vi "pic_step1.vi"() -> ()   [LabVIEW 2018]
uses:
  Device VIs/Verbal.vi
  <vilib>/Instr/_visa.llb/VISA Configure Serial Port (Instr).vi
panel:
  in  "结束":bool
  out "P3右":bool
  out "P2 右":bool
  out "P1 右":bool
  out "pic3Left":bool caption="0位"
  out "pic3Right":bool caption="限位"
  out "pic2Left":bool caption="0位"
  out "pic2Right":bool caption="限位"
  out "pic1Left":bool caption="0位"
  out "pic1Right":bool caption="限位"
  out "CH3 当前位置":i32
  in  "P3jog":bool caption="X jog"
  out "P3设定位置":i32
  in  "pic3位置":u16(ring) caption="位置" items=["位置0", "位置1", "位置2", "位置3"]
  in  "P3归0":bool
  in  "CH3启动":bool
  in  "CH3 运动步数":i32 caption="P3 步进"
  in  "Y 连续正转":bool
  in  "X连续反转":bool
  out "Yflag":bool
  out "0位":u8
  in  "P2 jog":bool caption="X jog"
  in  "P1jog":bool caption="X jog"
  in  "Zjog":bool caption="X jog"
  in  "Yjog":bool caption="X jog"
  in  "X jog":bool
  out "P2设定位置":i32
  out "P1设定位置":i32
  out "Z设定位置":i32
  out "Y设定位置":i32
  out "X设定位置":i32
  in  "pic2位置":u16(ring) caption="位置" items=["位置0", "位置1", "位置2", "位置3"]
  in  "pic1位置":u16(ring) caption="位置" items=["位置0", "位置1", "位置2", "位置3"]
  in  "Z轴位置":u16(ring) caption="位置" items=["位置0", "位置1", "位置2", "位置3"]
  in  "Y轴位置":u16(ring) caption="位置" items=["位置0", "位置1", "位置2", "位置3"]
  in  "X轴位置":u16(ring) caption="位置" items=["位置0", "位置1", "位置2", "位置3"]
  out "执行":bool
  in  "Z 归0":bool
  in  "Y 归0":bool
  in  "X 归0":bool
  out "当前位置":string[](array[string])
  in  "Z 连续反转":bool
  in  "Z 连续正转":bool
  in  "Y 连续反转":bool
  in  "X 连续正转":bool
  out "Z Left":bool caption="0位"
  out "Z Right":bool caption="限位"
  out "Y Left":bool caption="0位"
  out "Y Right":bool caption="限位"
  out "X Lift":bool caption="0位"
  out "X Right":bool caption="限位"
  in  "Z 启动":bool
  in  "Y 启动":bool
  in  "X 启动":bool
  in  "Step Z":i32 caption="Z 步进" min=-8388607 max=8388607
  in  "Step Y":i32 caption="Y 步进" min=-8388607 max=8388607
  in  "Step X":i32 caption="X 步进" min=-8388607 max=8388607
  in  "P2归0":bool
  in  "P1 归0":bool
  out "OK":bool
  in  "制动":bool
  in  "CH2启动":bool
  in  "CH1启动":bool
  in  "CH2 运动步数":i32 caption="P2 步进"
  in  "CH1 运动步数":i32 caption="P1 步进"
  out "CH2 当前位置":i32
  out "CH1 当前位置":i32
  out "状态":string
  out "error out":errorcluster
  # "X"
  # "Y"
  # "Z"
  # "P1"
  # "P2"
  # "P3"
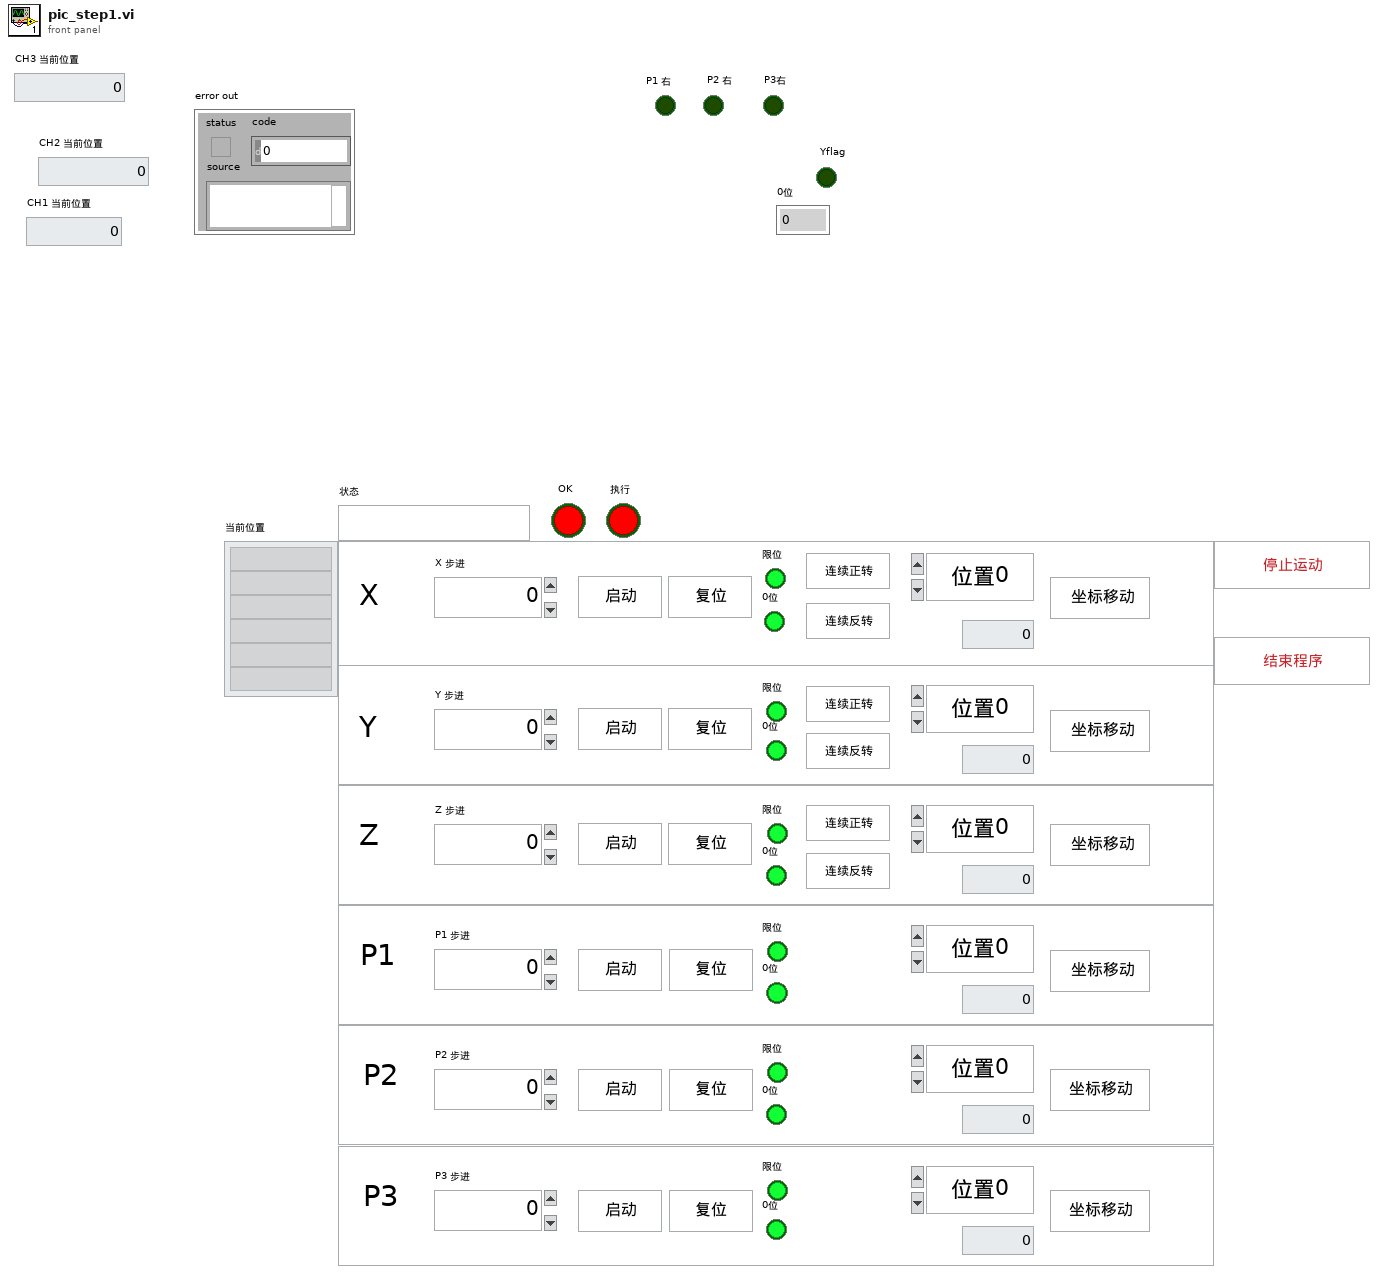
[diagram p1: front panel]
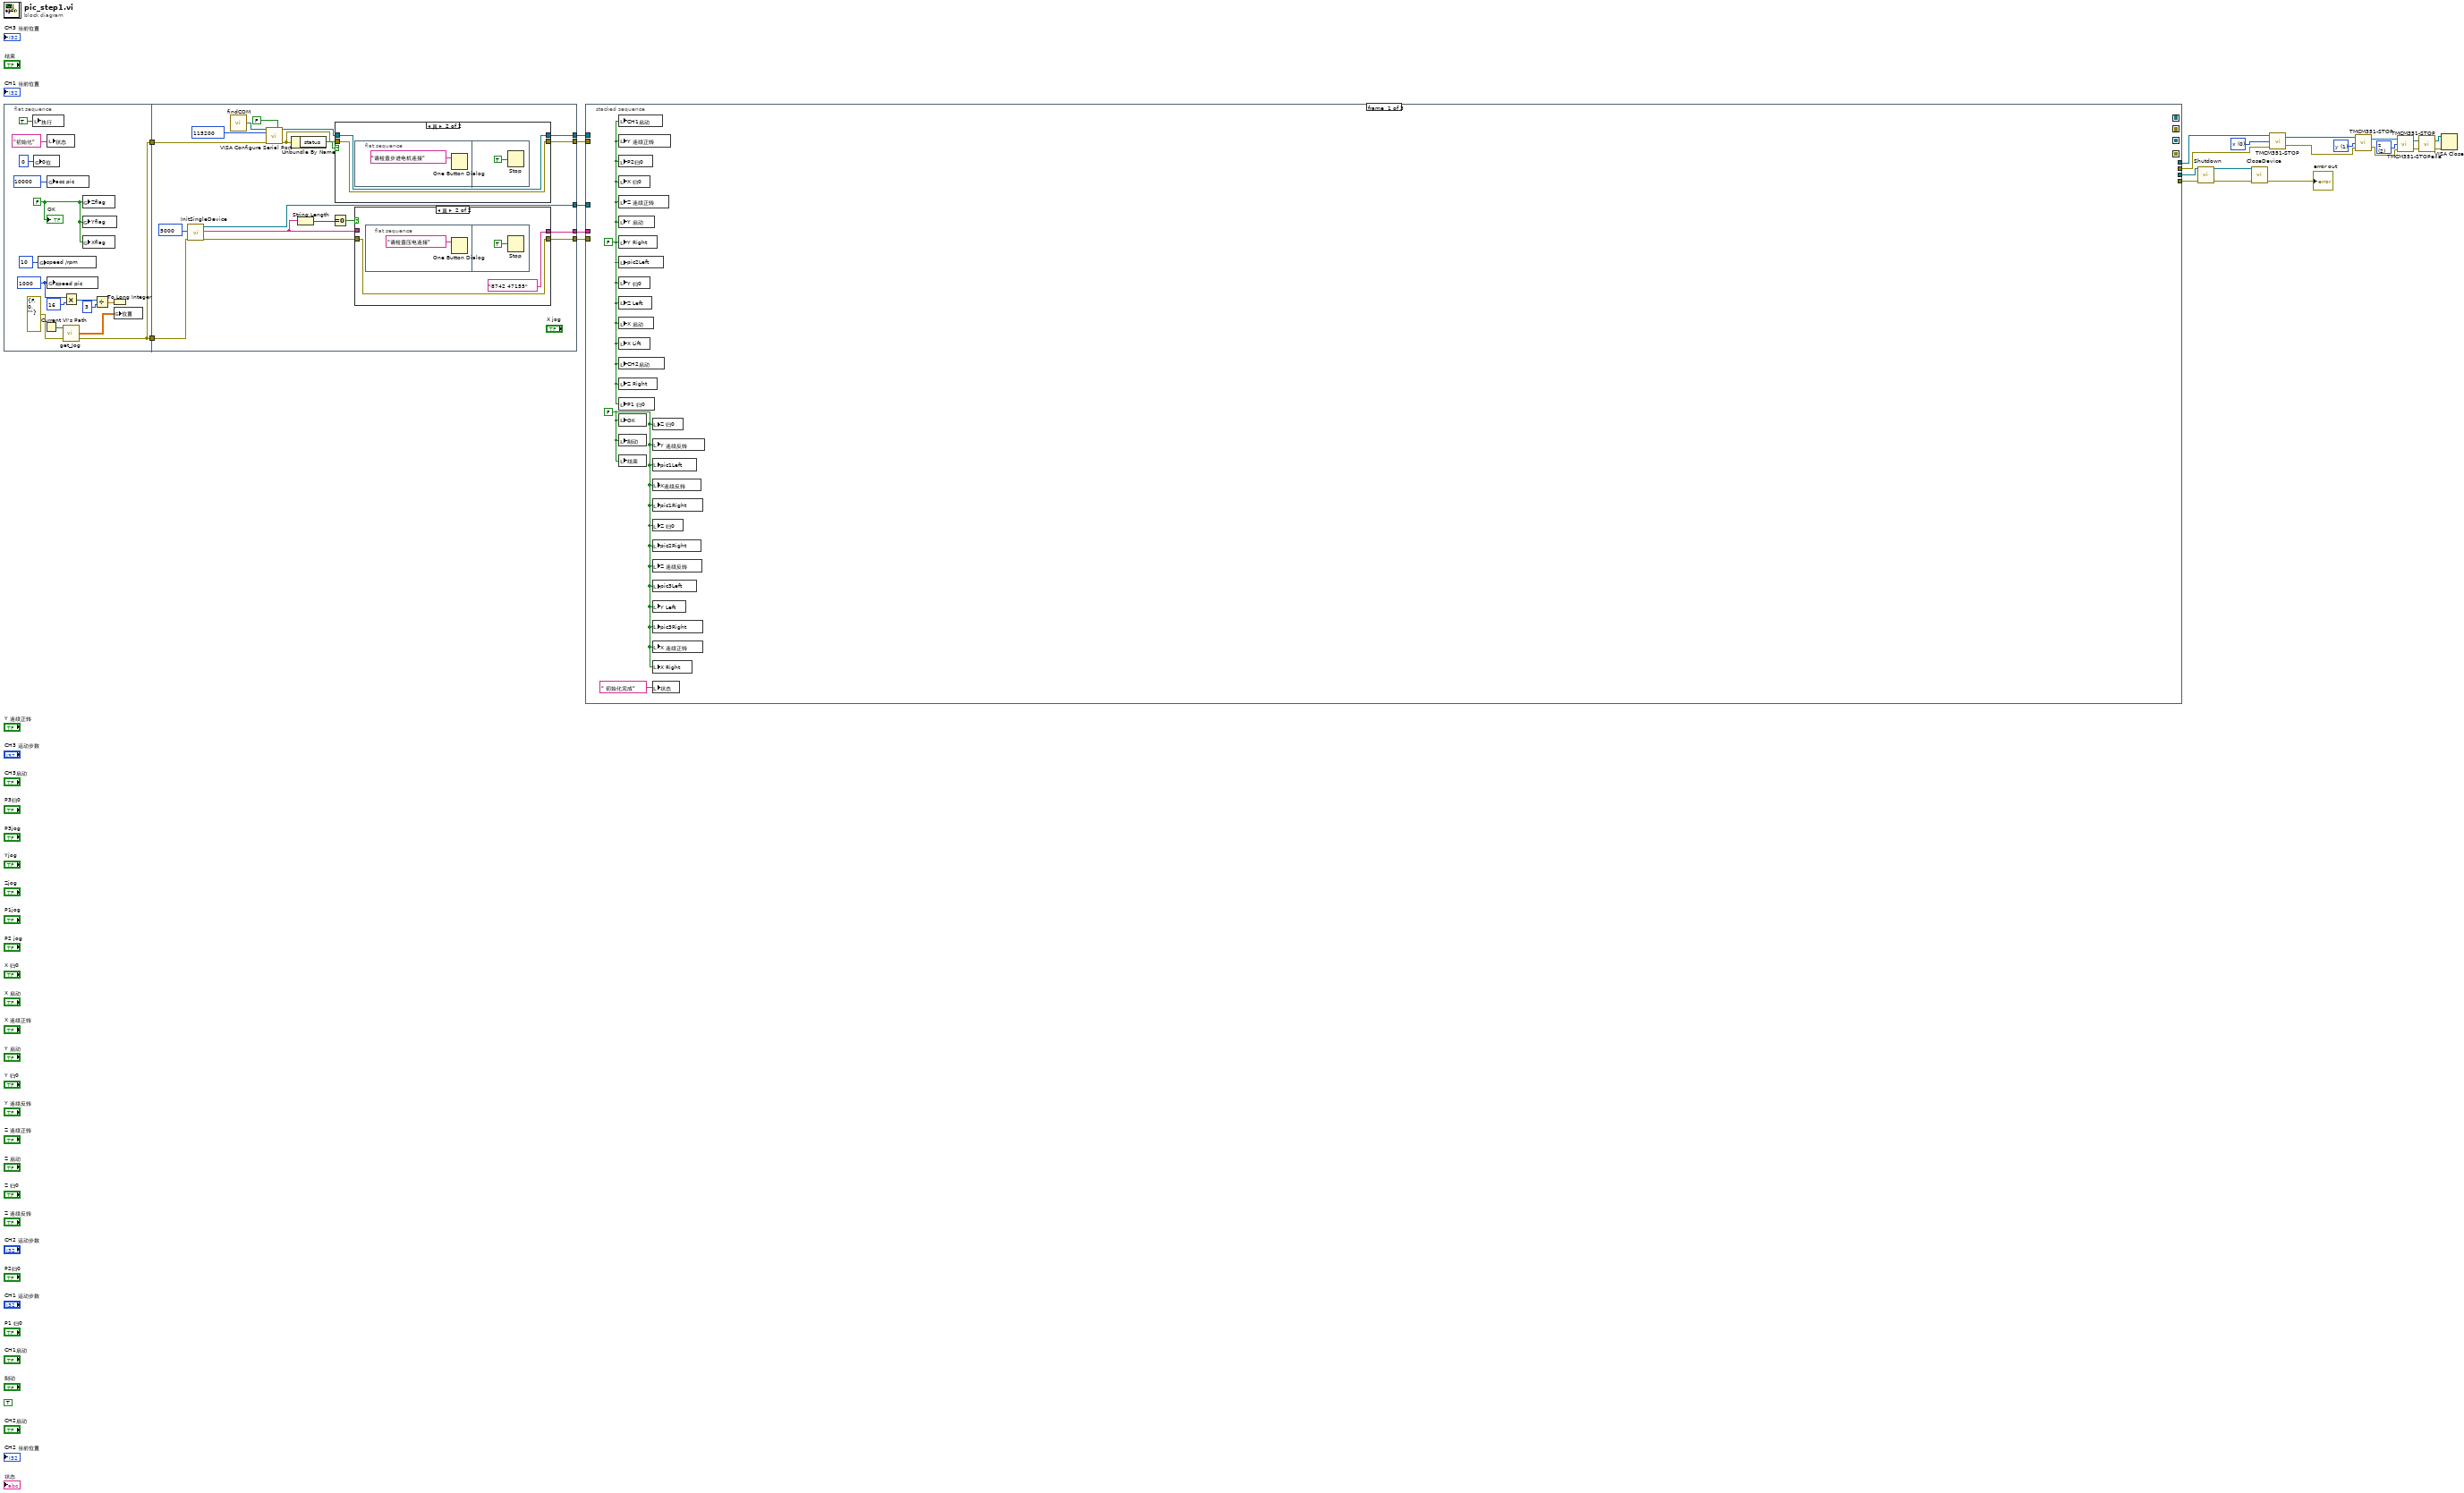
[diagram p0: block diagram]
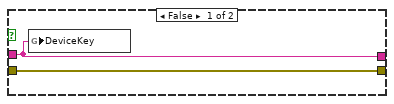
[diagram p2: hidden frame]
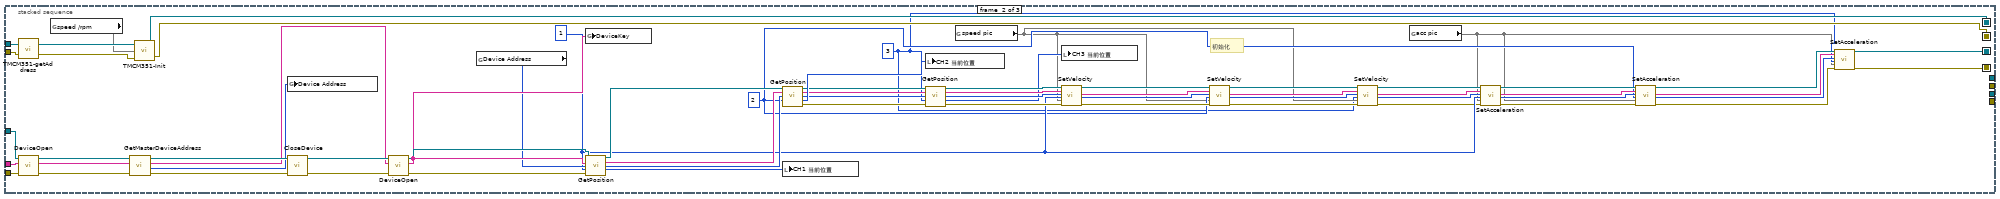
[diagram p4: hidden frame]
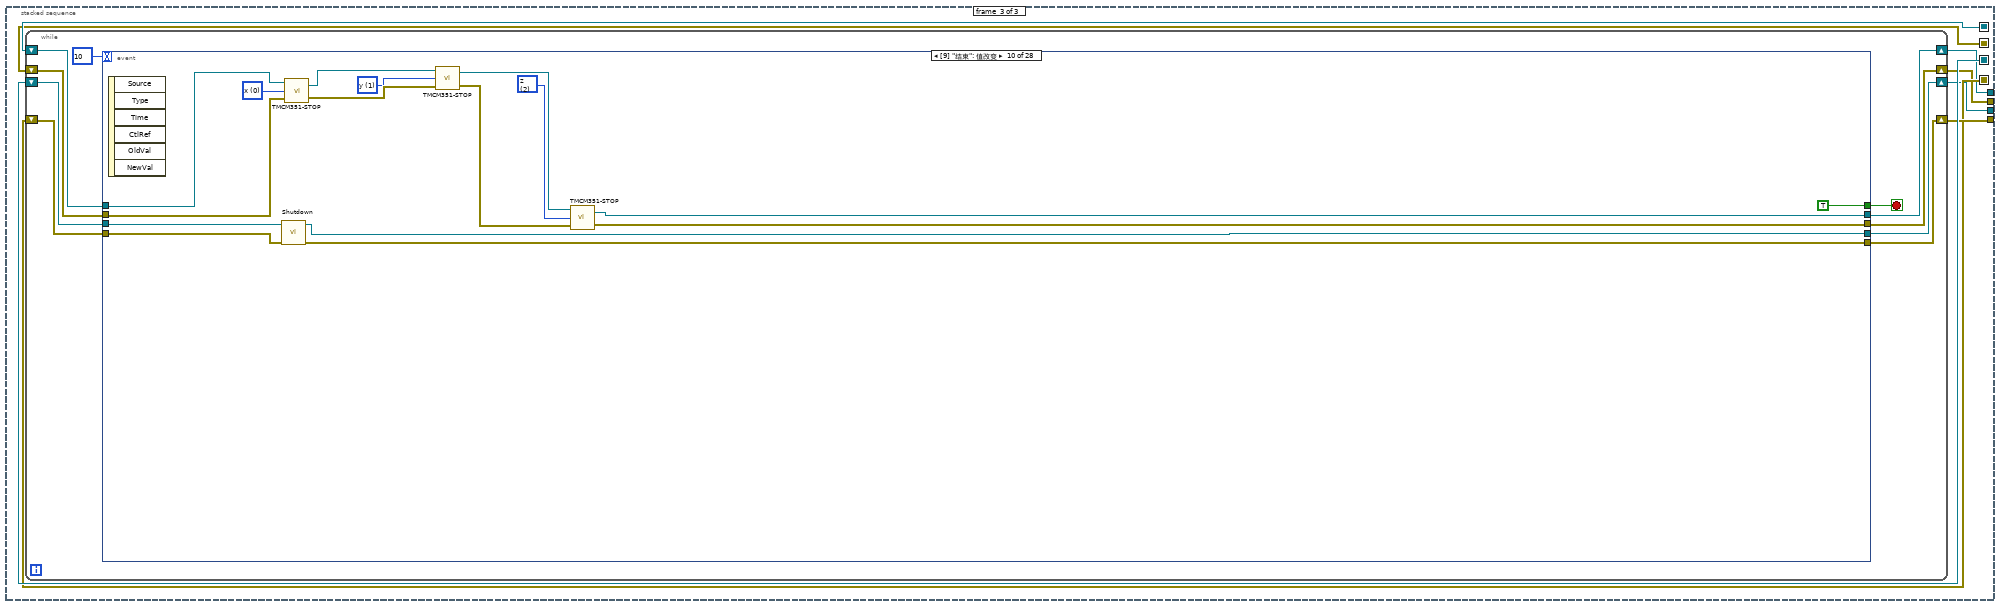
[diagram p5: hidden frame]
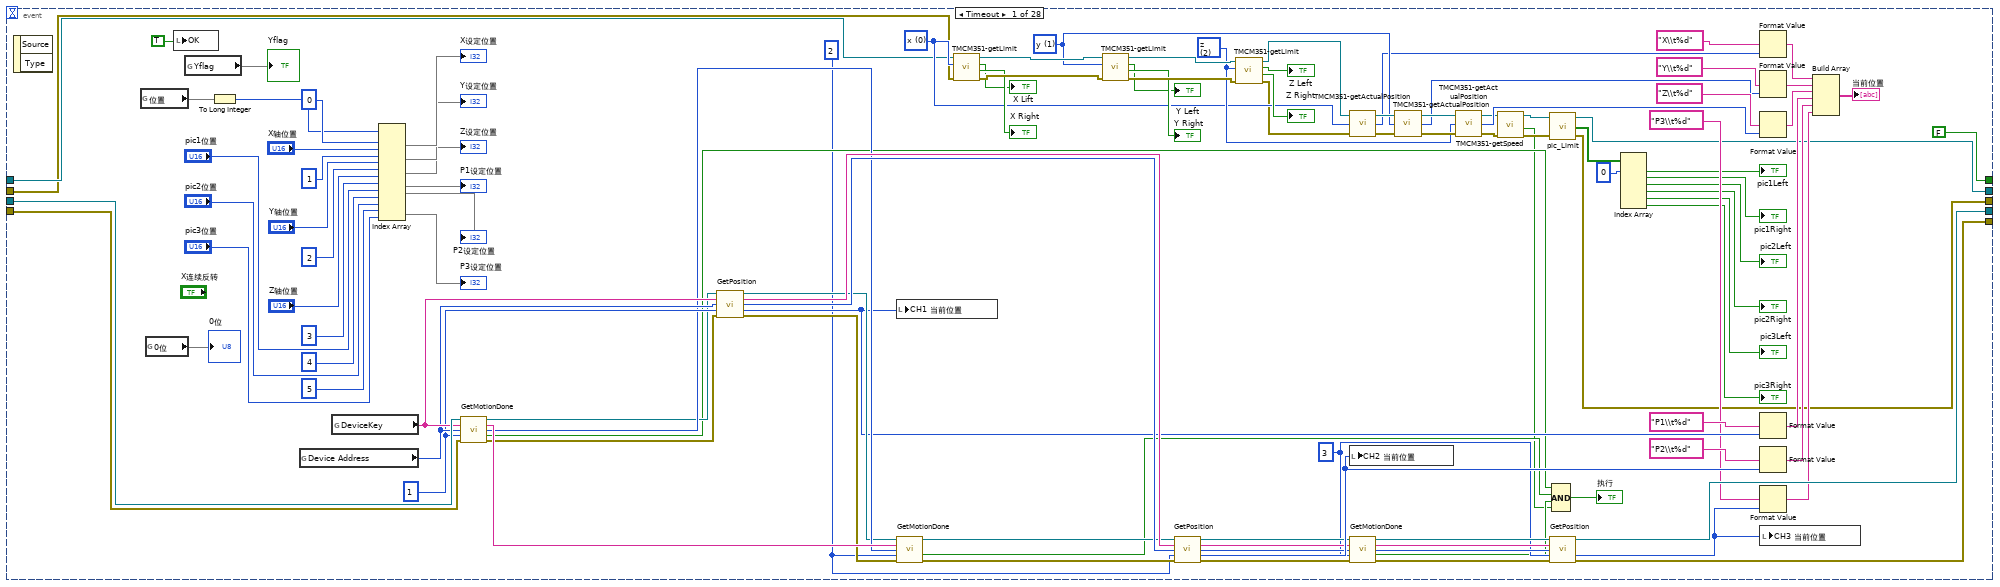
[diagram p6: hidden frame]
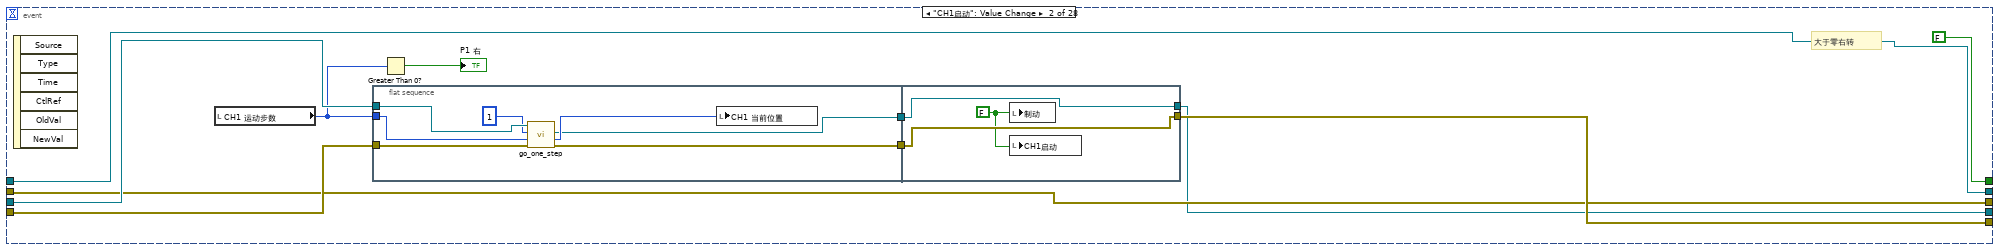
[diagram p7: hidden frame]
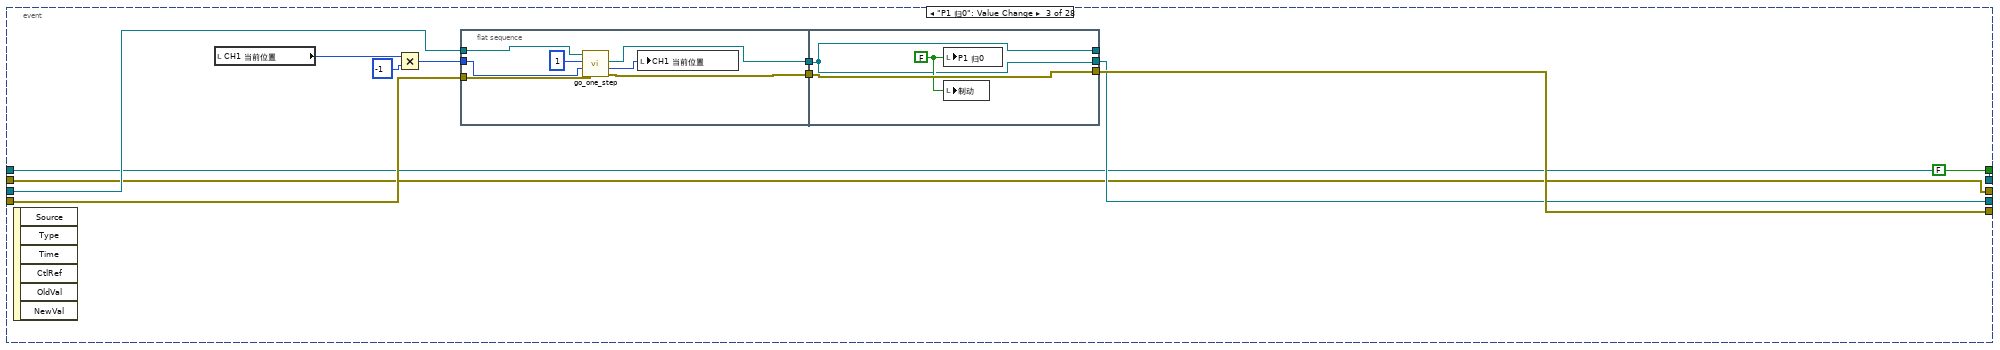
[diagram p8: hidden frame]
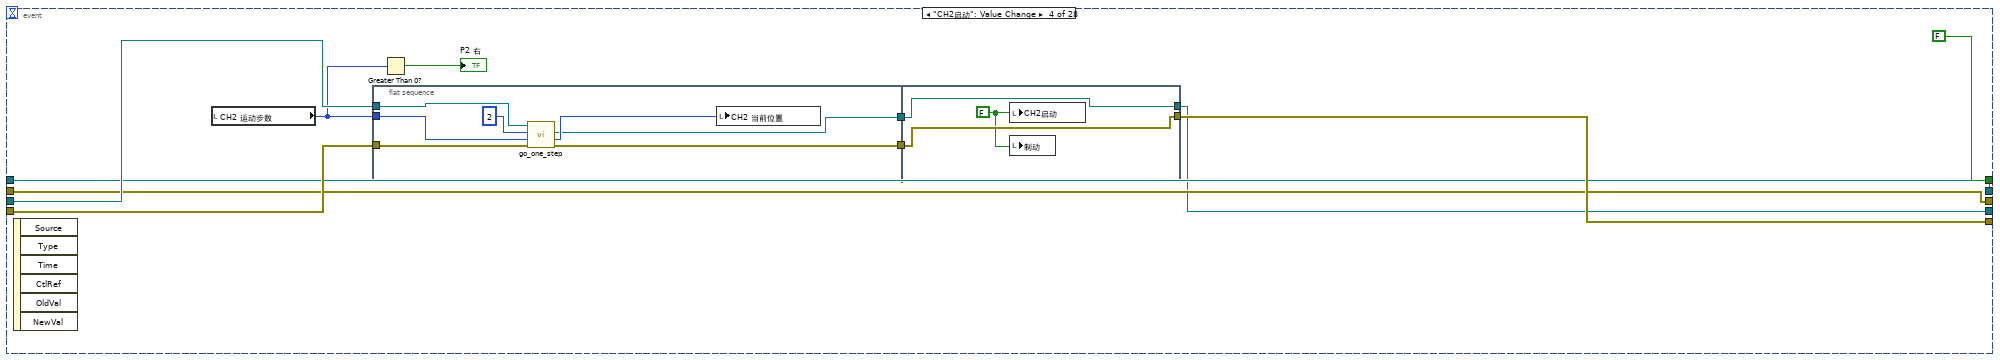
[diagram p9: hidden frame]
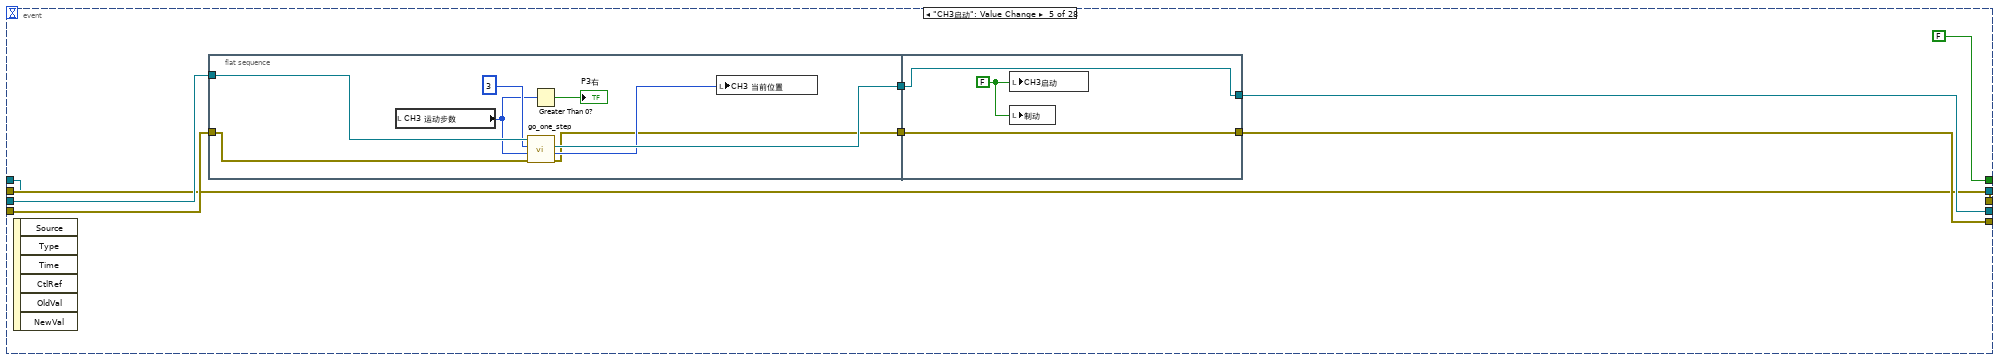
[diagram p10: hidden frame]
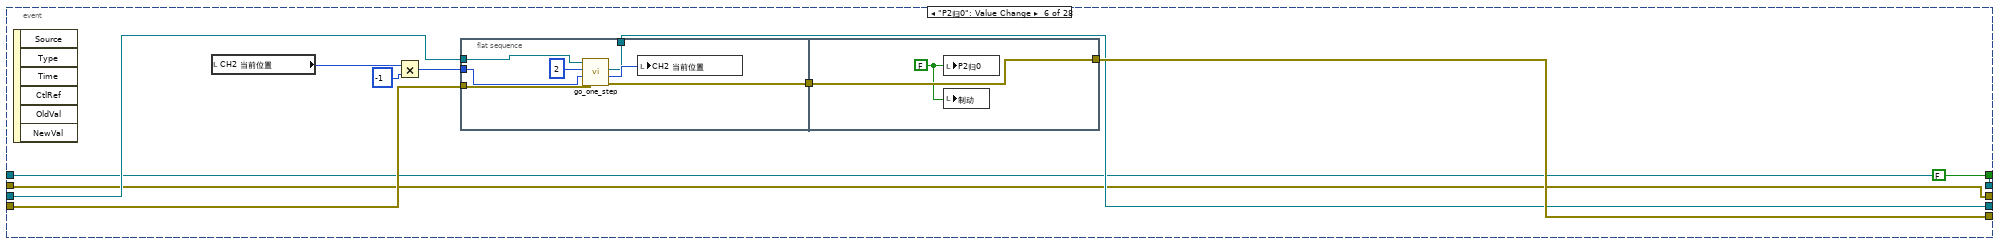
[diagram p11: hidden frame]
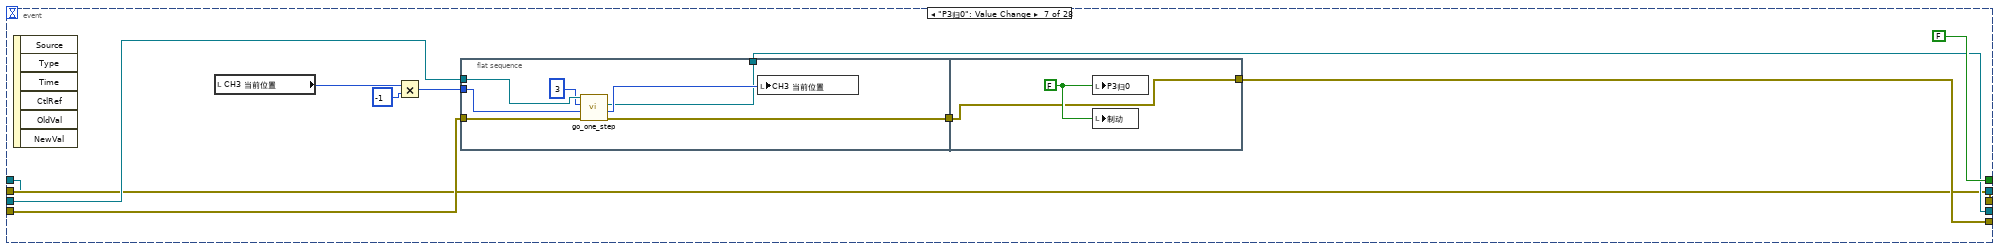
[diagram p12: hidden frame]
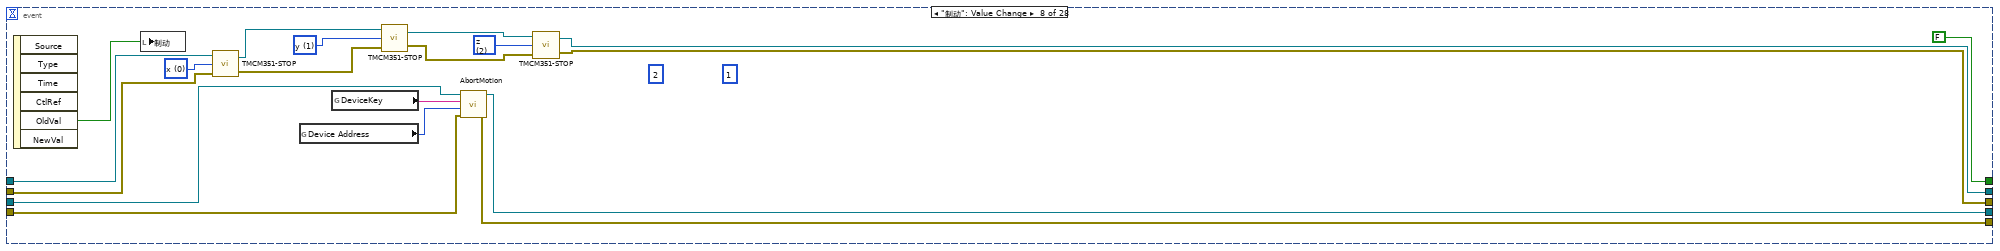
[diagram p13: hidden frame]
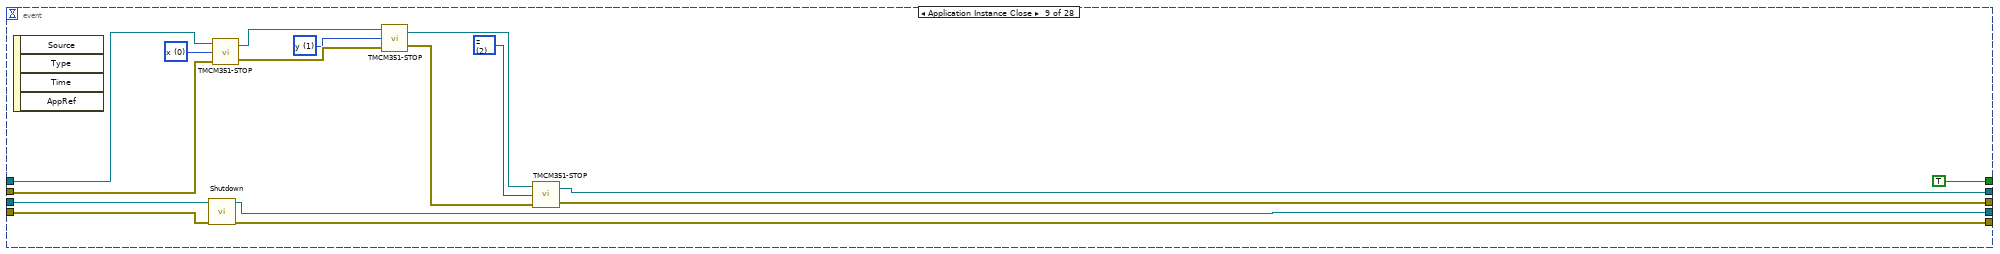
[diagram p14: hidden frame]
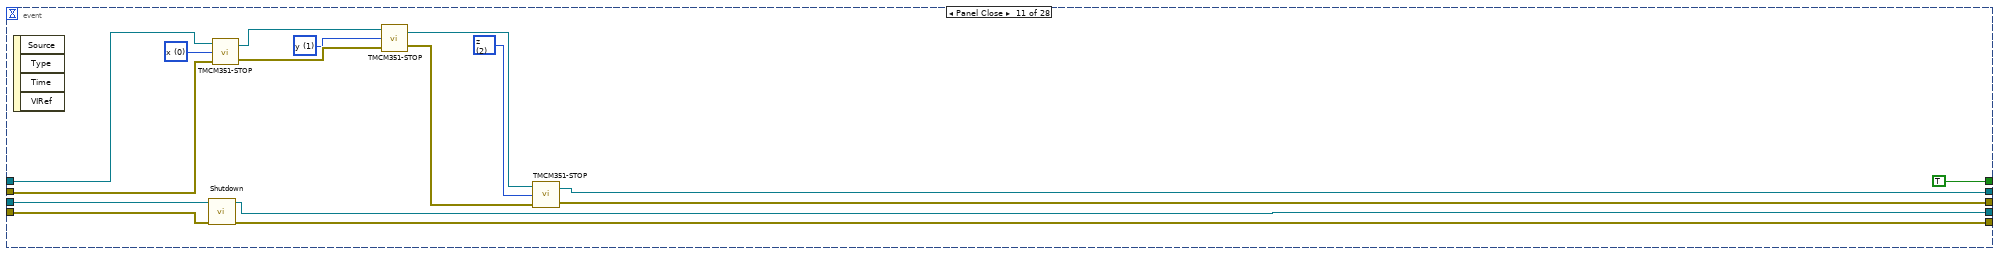
[diagram p15: hidden frame]
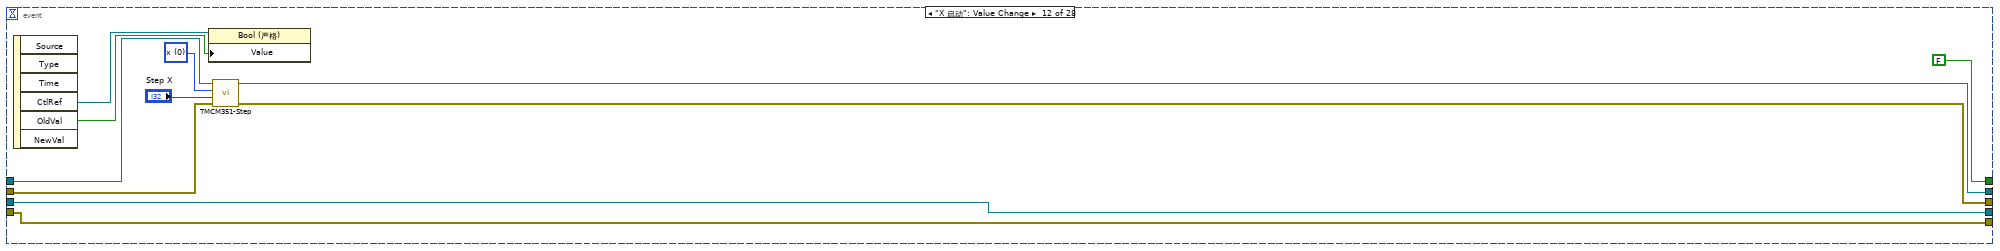
[diagram p16: hidden frame]
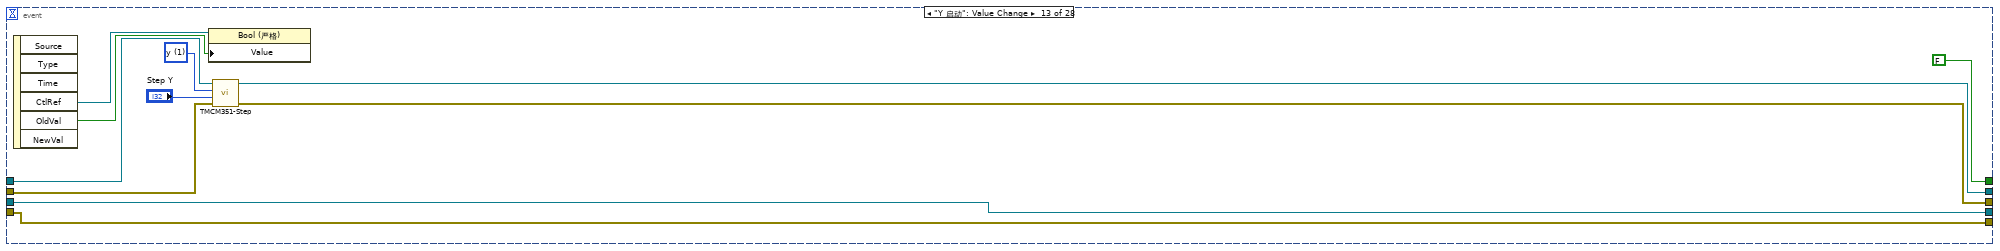
[diagram p17: hidden frame]
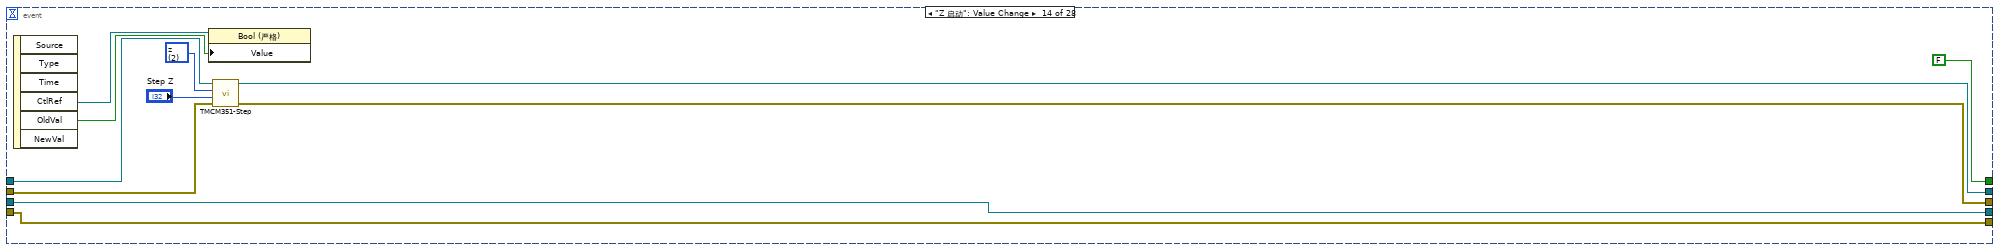
[diagram p18: hidden frame]
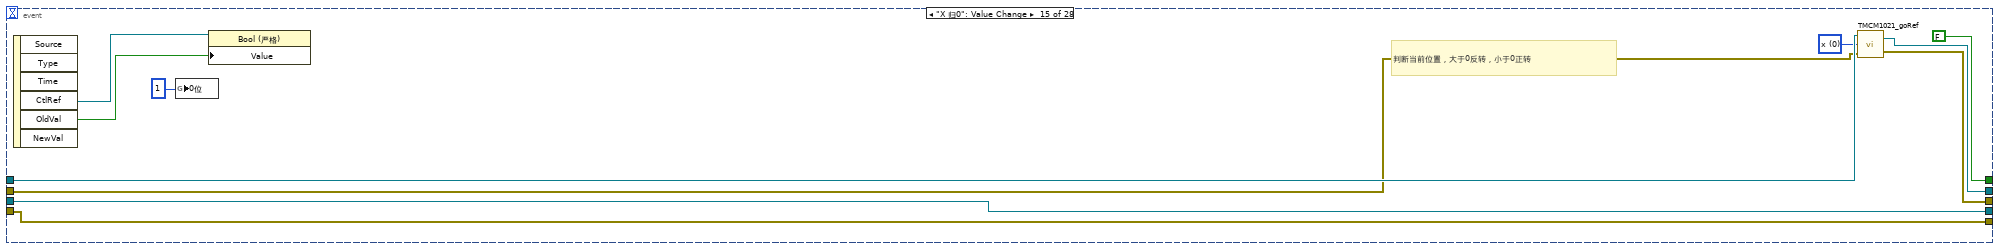
[diagram p19: hidden frame]
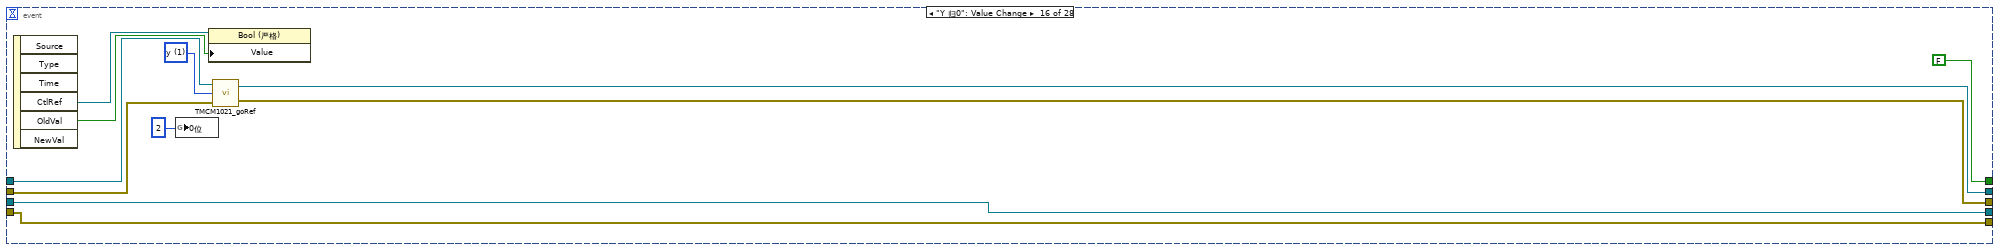
[diagram p20: hidden frame]
diagram:
  w10 = u8 2 items=["x", "y", "z"] ("motor")
  w11 = u8 1 items=["x", "y", "z"] ("motor")
  w12 = u8 0 items=["x", "y", "z"] ("motor")
  (unwired) TRUE
  n1 = flat-sequence {
    tunnel: [w30] -> w2
    tunnel: [w30] -> w1
    tunnel: [w48] -> w25
    tunnel: [w46] -> w24
    tunnel: [w52] -> w23
    tunnel: [w51] -> w22
    tunnel: [w50] -> w21
    tunnel: w2 -> [w49]
    tunnel: w1 -> [w44]
    frame #0 {
      w27 = FALSE ("OK")
      w35 = 1000 ("speed pic")
      n2 = local write "执行"(TRUE ("执行")) -> ()
      n3 = global write "Verbal.vi" "0位"(u8 0 ("0位")) -> ()
      n4 = global write "Verbal.vi" "speed /rpm"(10 ("speed step")) -> ()
      n5 = Current VI's Path() -> (path=w32:path)
      n6 = local write "状态"("初始化" ("状态")) -> ()
      n7 = global write "Verbal.vi" "acc pic"(10000 ("acc pic")) -> ()
      n8 = global write "Verbal.vi" "speed pic"(w35) -> ()
      n9 = call "get_Jog.vi"("error in (no error)"=errorcluster {"status"=FALSE, "code"=0, "source"=""}, "路径"=w32) -> ("error out"=w30:errorcluster, "位置out"=w29:dbl[][])  [unwired: 2 in]
      n10 = Multiply(x=w35, y=u16 16) -> (x*y=w37:i32)
      n11 = global write "Verbal.vi" "Zflag"(w27) -> ()
      n12 = global write "Verbal.vi" "Yflag"(w27) -> ()
      n13 = global write "Verbal.vi" "Xflag"(w27) -> ()
      n14 = Divide(x=w37, y=u16 3) -> (x/y=w34:dbl)
      n15 = To Long Integer(number=w34) -> ()  [unwired: 1 out]
      n16 = global write "Verbal.vi" "位置"(w29) -> ()
      "OK" <- w27
    }
    frame #1 {
      n17 = call "InitSingleDevice.vi"("error in (no error)"=w44, "msecDelayForDiscovery"=5000) -> ("error out"=w45:errorcluster, "DeviceKey Out"=w42:string, "CmdLib Out"=w46:refnum<k24>)  [unwired: 3 in]
      n18 = call "findCOM.vi"() -> ("VISA resource out"=w56:refnum<visa-resource-name>)  [unwired: 1 in]
      n19 = call-poly "VISA Configure Serial Port"("VISA resource name"=w56, "Enable Termination\nChar (T)"=FALSE ("Enable Termination\nChar (T)"), "baud rate (9600)"=u32 115200, "error in (no error)"=w49) -> ("VISA resource name out"=w55:refnum<visa-resource-name>, "error out"=w53:errorcluster)  [unwired: 10 in]
      n20 = Unbundle By Name(w53) -> ("status"=w54:bool)
      n21 = String Length(string=w42) -> (length=w43:i32)
      n22 = Equal To 0?(x=w43) -> (x = 0?=w41:bool)
      n23 = case shown="真" w54 {
        tunnel: w55 -> [w66 w68]
        tunnel: w53 -> [w65 w67]
        tunnel: [w66 w68] -> w50
        tunnel: [w65 w67] -> w51
        frame False {
        }
        frame True {
          n24 = flat-sequence {
            frame #0 {
              n25 = One Button Dialog(message="请检查步进电机连接" ("消息")) -> ()  [unwired: 1 in, 1 out]
            }
            frame #1 {
              n26 = Stop(stop? (T)=TRUE ("停止？(T)")) -> ()
            }
          }
        }
      }
      n27 = case shown="真" w41 {
        tunnel: [w60 w62] -> w52
        tunnel: w45 -> [w60 w62]
        tunnel: [w59 "8742 47155" ("Message")] -> w48
        tunnel: w42 -> [w59 _]
        frame False {
          n28 = global write "Verbal.vi" "DeviceKey"(w59) -> ()
        }
        frame True {
          n29 = flat-sequence {
            frame #0 {
              n30 = One Button Dialog(message="请检查压电连接" ("消息")) -> ()  [unwired: 1 in, 1 out]
            }
            frame #1 {
              n31 = Stop(stop? (T)=TRUE ("停止？(T)")) -> ()
            }
          }
        }
      }
    }
  }
  n32 = stacked-sequence {
    seq-local: [_ w85 _] -> [_ _ w145]
    seq-local: [_ w84 _] -> [_ _ w143]
    seq-local: [_ w135 _] -> [_ _ w142]
    seq-local: [_ w134 _] -> [_ _ w141]
    tunnel: w25 -> [_ w77 _]
    tunnel: [_ _ w144] -> w3
    tunnel: w24 -> [_ w81 _]
    tunnel: w23 -> [_ w79 _]
    tunnel: w22 -> [_ w137 _]
    tunnel: w21 -> [_ w136 _]
    tunnel: [_ _ w140] -> w14
    tunnel: [_ _ w139] -> w13
    tunnel: [_ _ w138] -> w4
    frame #0 {
      w72 = FALSE
      w71 = FALSE
      n33 = local write "CH1启动"(w72) -> ()
      n34 = local write "Y 连续正转"(w72) -> ()
      n35 = local write "P2归0"(w72) -> ()
      n36 = local write "X 归0"(w72) -> ()
      n37 = local write "Z 连续正转"(w72) -> ()
      n38 = local write "Y 启动"(w72) -> ()
      n39 = local write "Y Right"(w72) -> ()
      n40 = local write "pic2Left"(w72) -> ()
      n41 = local write "Y 归0"(w72) -> ()
      n42 = local write "Z Left"(w72) -> ()
      n43 = local write "X 启动"(w72) -> ()
      n44 = local write "X Lift"(w72) -> ()
      n45 = local write "CH2启动"(w72) -> ()
      n46 = local write "Z Right"(w72) -> ()
      n47 = local write "P1 归0"(w72) -> ()
      n48 = local write "OK"(w71) -> ()
      n49 = local write "制动"(w71) -> ()
      n50 = local write "结束"(w71) -> ()
      n51 = local write "Z 归0"(w71) -> ()
      n52 = local write "Y 连续反转"(w71) -> ()
      n53 = local write "pic1Left"(w71) -> ()
      n54 = local write "X连续反转"(w71) -> ()
      n55 = local write "pic1Right"(w71) -> ()
      n56 = local write "Z 归0"(w71) -> ()
      n57 = local write "pic2Right"(w71) -> ()
      n58 = local write "Z 连续反转"(w71) -> ()
      n59 = local write "pic3Left"(w71) -> ()
      n60 = local write "Y Left"(w71) -> ()
      n61 = local write "pic3Right"(w71) -> ()
      n62 = local write "X 连续正转"(w71) -> ()
      n63 = local write "X Right"(w71) -> ()
      n64 = local write "状态"(" 初始化完成" ("Message")) -> ()
    }
    frame #1 {
      w87 = 3 ("Motor")
      w101 = 2 ("Motor")
      w102 = 1 ("Motor")
      # "初始化"
      n65 = call "TMCM351-getAddress.vi"("错误输入"=w137, "com in"=w136) -> ("错误输出"=w118:errorcluster, "com out"=w113:refnum<visa-resource-name>)
      n66 = call "DeviceOpen.vi"("error in (no error)"=w79, "DeviceKey In"=w77, "CmdLib In"=w81) -> ("error out"=w82:errorcluster, "DeviceKey Out"=w76:string, "CmdLib Out"=w83:refnum<k24>)  [unwired: 2 in]
      n67 = global read "Verbal.vi" "speed /rpm"() -> (w112)
      n68 = call "GetMasterDeviceAddress.vi"("error in (no error)"=w82, "DeviceKey In"=w76, "CmdLib In"=w83) -> ("error out"=w78:errorcluster, "Device Address"=w75:i32, "DeviceKey Out"=w74:string, "CmdLib Out"=w80:refnum<k24>)  [unwired: 1 in]
      n69 = call "TMCM351-Init.vi"("错误输入"=w118, "Speed /rpm"=w112, "com in"=w113) -> ("错误输出"=w134:errorcluster, "com out"=w135:refnum<visa-resource-name>)
      n70 = global write "Verbal.vi" "Device Address"(w75) -> ()
      n71 = call "CloseDevice.vi"("error in"=w78, "CmdLib In"=w80) -> ("error out"=w132:errorcluster, "CmdLib Out"=w133:refnum<k24>)  [unwired: 8 in]
      n72 = call "DeviceOpen.vi"("error in (no error)"=w132, "DeviceKey In"=w74, "CmdLib In"=w133) -> ("error out"=w128:errorcluster, "DeviceKey Out"=w130:string, "CmdLib Out"=w131:refnum<k24>)  [unwired: 2 in]
      n73 = global read "Verbal.vi" "Device Address"() -> (w129:i32)
      n74 = global write "Verbal.vi" "DeviceKey"(w130) -> ()
      n75 = call "GetPosition.vi"("CmdLib In"=w131, "DeviceKey In"=w130, "Device Address In"=w129, "Motor"=w102, "error in (no error)"=w128) -> ("CmdLib Out"=w126:refnum<k24>, "DeviceKey Out"=w125:string, "Device Address Out"=w124:i32, "Position"=w127:i32)  [unwired: 6 in, 1 out]
      n76 = call "GetPosition.vi"("CmdLib In"=w126, "DeviceKey In"=w125, "Device Address In"=w124, "Motor"=w101) -> ("CmdLib Out"=w111:refnum<k24>, "DeviceKey Out"=w110:string, "Device Address Out"=w109:i32, "Position"=w123:i32, "error out"=w108:errorcluster)  [unwired: 7 in]
      n77 = local write "CH1 当前位置"(w127) -> ()
      n78 = local write "CH2 当前位置"(w123) -> ()
      n79 = call "GetPosition.vi"("CmdLib In"=w111, "DeviceKey In"=w110, "Device Address In"=w109, "Motor"=w87, "error in (no error)"=w108) -> ("CmdLib Out"=w106:refnum<k24>, "DeviceKey Out"=w105:string, "Device Address Out"=w104:i32, "Position"=w103:i32, "error out"=w107:errorcluster)  [unwired: 6 in]
      n80 = global read "Verbal.vi" "speed pic"() -> (w97)
      n81 = local write "CH3 当前位置"(w103) -> ()
      n82 = call "SetVelocity.vi"("CmdLib In"=w106, "DeviceKey In"=w105, "Device Address In"=w104, "Motor"=w102, "Steps Per Sec"=w97, "error in (no error)"=w107) -> ("CmdLib Out"=w122:refnum<k24>, "DeviceKey Out"=w121:string, "Device Address Out"=w120:i32, "error out"=w119:errorcluster)  [unwired: 10 in]
      n83 = call "SetVelocity.vi"("CmdLib In"=w122, "DeviceKey In"=w121, "Device Address In"=w120, "Motor"=w101, "Steps Per Sec"=w97, "error in (no error)"=w119) -> ("CmdLib Out"=w100:refnum<k24>, "DeviceKey Out"=w99:string, "Device Address Out"=w98:i32, "error out"=w96:errorcluster)  [unwired: 10 in]
      n84 = call "SetVelocity.vi"("CmdLib In"=w100, "DeviceKey In"=w99, "Device Address In"=w98, "Motor"=w87, "Steps Per Sec"=w97, "error in (no error)"=w96) -> ("CmdLib Out"=w95:refnum<k24>, "DeviceKey Out"=w94:string, "Device Address Out"=w93:i32, "error out"=w92:errorcluster)  [unwired: 10 in]
      n85 = global read "Verbal.vi" "acc pic"() -> (w86)
      n86 = call "SetAcceleration.vi"("CmdLib In"=w95, "DeviceKey In"=w94, "Device Address In"=w93, "Motor"=w102, "Steps Per Sec 2"=w86, "error in (no error)"=w92) -> ("CmdLib Out"=w117:refnum<k24>, "DeviceKey Out"=w116:string, "Device Address Out"=w115:i32, "error out"=w114:errorcluster)  [unwired: 10 in]
      n87 = call "SetAcceleration.vi"("CmdLib In"=w117, "DeviceKey In"=w116, "Device Address In"=w115, "Motor"=w101, "Steps Per Sec 2"=w86, "error in (no error)"=w114) -> ("CmdLib Out"=w91:refnum<k24>, "DeviceKey Out"=w90:string, "Device Address Out"=w89:i32, "error out"=w88:errorcluster)  [unwired: 10 in]
      n88 = call "SetAcceleration.vi"("CmdLib In"=w91, "DeviceKey In"=w90, "Device Address In"=w89, "Motor"=w87, "Steps Per Sec 2"=w86, "error in (no error)"=w88) -> ("CmdLib Out"=w85:refnum<k24>, "error out"=w84:errorcluster)  [unwired: 10 in, 2 out]
    }
    frame #2 {
      n89 = while {
        shift-right: [w153] -> w144
        shift-left: w143 -> [w151]
        shift-right: [w150] -> w138
        shift-left: w145 -> [w154]
        shift-right: [w149] -> w140
        shift-left: w142 -> [w147]
        shift-right: [w148] -> w139
        shift-left: w141 -> [w146]
        stop <- w152 stop-if-true
        n90 = event shown="[9] \"结束\": 值改变" {
          selector: _ -> [_ _ _ _ _ _ _ _ _ _ _ _ _ _ _ _ _ _ _ _ _ _ _ _ _ _ _ _]
          dyn-events: _ -> [_ _ _ _ _ _ _ _ _ _ _ _ _ _ _ _ _ _ _ _ _ _ _ _ _ _ _ _]
          timeout: 10 -> [_ _ _ _ _ _ _ _ _ _ _ _ _ _ _ _ _ _ _ _ _ _ _ _ _ _ _ _]
          tunnel: w154 -> [w262 w276 w295 w319 w338 w357 w376 w406 w424 w431 w456 w461 w474 w485 w500 w511 w522 w525 w537 w549 w561 w573 w585 w597 w608 w619 w638 w651]
          tunnel: w151 -> [w221 w275 w294 w317 w337 w356 w375 w407 w423 w430 w455 w460 w473 w484 w499 w510 w521 w524 w536 w548 w560 w572 w584 w596 w607 w618 w633 w646]
          tunnel: [w174 w274 w292 w318 w335 w355 w374 w392 w422 w426 w454 w460 w473 w484 w499 w510 w521 w524 w536 w548 w560 w572 w584 w596 w607 w618 w631 w644] -> w153
          tunnel: [FALSE FALSE FALSE FALSE FALSE FALSE FALSE FALSE TRUE TRUE TRUE FALSE FALSE FALSE FALSE FALSE FALSE FALSE FALSE FALSE FALSE FALSE FALSE FALSE FALSE FALSE FALSE FALSE] -> w152
          tunnel: w147 -> [w204 w271 w288 w314 w333 w351 w370 w404 w413 w435 w444 w466 w477 w489 w494 w505 w517 w534 w543 w555 w567 w579 w591 w603 w614 w625 w630 w643]
          tunnel: w146 -> [w203 w270 w287 w313 w334 w350 w371 w403 w412 w432 w443 w465 w476 w487 w491 w504 w516 w533 w542 w554 w566 w578 w590 w602 w613 w624 w629 w642]
          tunnel: [w175 w268 w289 w311 w336 w352 w372 w391 w409 w427 w452 w461 w474 w485 w500 w511 w522 w525 w537 w549 w561 w573 w585 w597 w608 w619 w632 w645] -> w150
          tunnel: [w168 w271 w288 w314 w333 w351 w370 w395 w411 w429 w442 w463 w472 w483 w493 w502 w514 w529 w541 w553 w565 w577 w589 w601 w610 w621 w630 w643] -> w149
          tunnel: [w167 w270 w287 w313 w334 w350 w371 w394 w410 w428 w441 w462 w471 w482 w492 w501 w513 w528 w540 w552 w564 w576 w588 w600 w609 w620 w629 w642] -> w148
          event Timeout {
            w177 = 3 ("Motor")
            w237 = u8 2 items=["x", "y", "z"] ("motor")
            w224 = u8 1 items=["x", "y", "z"] ("motor")
            w225 = u8 0 items=["x", "y", "z"] ("motor")
            w178 = 2 ("Motor")
            w259 = 1 ("Motor")
            n91 = event-data() -> ()  [unwired: 1 in, 2 out]
            n92 = global read "Verbal.vi" "位置"() -> (w199)
            n93 = global read "Verbal.vi" "0位"() -> (→"0位")
            n94 = local write "OK"(TRUE ("等待指令")) -> ()
            n95 = global read "Verbal.vi" "Yflag"() -> (→"Yflag")
            n96 = To Long Integer(number=w199) -> (32bit integer=w198:i32)
            n97 = global read "Verbal.vi" "Device Address"() -> (w260:i32)
            n98 = global read "Verbal.vi" "DeviceKey"() -> (w261:string)
            n99 = Index Array(array=w198, index (row) #1=0 ("索引 (行)"), index (col) #1="X轴位置", index (row) #2=1 ("索引 (行)"), index (col) #2="Y轴位置", index (row) #3=2 ("索引 (行)"), index (col) #3="Z轴位置", index (row) #4=3 ("索引 (行)"), index (col) #4="pic1位置", index (row) #5=4 ("索引 (行)"), index (col) #5="pic2位置", index (row) #6=5 ("索引 (行)"), index (col) #6="pic3位置") -> (element #1=→"X设定位置", element #2=→"Y设定位置", element #3=→"Z设定位置", element #4=→"P1设定位置", element #5=→"P2设定位置", element #6=→"P3设定位置")
            n100 = call "GetMotionDone.vi"("CmdLib In"=w262, "DeviceKey In"=w261, "Device Address In"=w260, "Motor"=w259, "error in (no error)"=w221) -> ("CmdLib Out"=w235:refnum<k24>, "DeviceKey Out"=w258:string, "Device Address Out"=w257:i32, "Is Motion Done"=w223:bool, "error out"=w236:errorcluster)  [unwired: 6 in]
            n101 = call "GetPosition.vi"("CmdLib In"=w235, "DeviceKey In"=w261, "Device Address In"=w260, "Motor"=w259, "error in (no error)"=w236) -> ("CmdLib Out"=w234:refnum<k24>, "DeviceKey Out"=w265:string, "Device Address Out"=w264:i32, "Position"=w227:i32, "error out"=w233:errorcluster)  [unwired: 6 in]
            n102 = local write "CH1 当前位置"(w227) -> ()
            n103 = call "GetMotionDone.vi"("CmdLib In"=w234, "DeviceKey In"=w258, "Device Address In"=w257, "Motor"=w178, "error in (no error)"=w233) -> ("CmdLib Out"=w232:refnum<k24>, "Is Motion Done"=w222:bool, "error out"=w231:errorcluster)  [unwired: 6 in, 2 out]
            n104 = call "TMCM351-getLimit.vi"("错误输入"=w203, "motor"=w225, "com in"=w204) -> ("错误输出"=w240:errorcluster, "right limit"=→"X Right":bool, "left limit"=→"X Lift":bool, "com out"=w241:refnum<visa-resource-name>)  [unwired: 1 in]
            n105 = call "TMCM351-getLimit.vi"("错误输入"=w240, "motor"=w224, "com in"=w241) -> ("错误输出"=w238:errorcluster, "right limit"=→"Y Right":bool, "left limit"=→"Y Left":bool, "com out"=w239:refnum<visa-resource-name>)  [unwired: 1 in]
            n106 = call "GetPosition.vi"("CmdLib In"=w232, "DeviceKey In"=w265, "Device Address In"=w264, "Motor"=w178, "error in (no error)"=w231) -> ("CmdLib Out"=w181:refnum<k24>, "DeviceKey Out"=w180:string, "Device Address Out"=w179:i32, "Position"=w226:i32, "error out"=w176:errorcluster)  [unwired: 6 in]
            n107 = call "TMCM351-getLimit.vi"("错误输入"=w238, "motor"=w237, "com in"=w239) -> ("错误输出"=w196:errorcluster, "right limit"=→"Z Right":bool, "left limit"=→"Z Left":bool, "com out"=w197:refnum<visa-resource-name>)  [unwired: 1 in]
            n108 = call "TMCM351-getActualPosition.vi"("错误输入"=w196, "motor"=w225, "com in"=w197) -> ("错误输出"=w255:errorcluster, "Pisotion"=w194:i32, "com out"=w256:refnum<visa-resource-name>)
            n109 = local write "CH2 当前位置"(w226) -> ()
            n110 = call "GetMotionDone.vi"("CmdLib In"=w181, "DeviceKey In"=w180, "Device Address In"=w179, "Motor"=w177, "error in (no error)"=w176) -> ("CmdLib Out"=w185:refnum<k24>, "DeviceKey Out"=w184:string, "Device Address Out"=w183:i32, "Is Motion Done"=w158:bool, "error out"=w182:errorcluster)  [unwired: 6 in]
            n111 = call "TMCM351-getActualPosition.vi"("错误输入"=w255, "motor"=w224, "com in"=w256) -> ("错误输出"=w253:errorcluster, "Pisotion"=w195:i32, "com out"=w254:refnum<visa-resource-name>)
            n112 = call "TMCM351-getActualPosition.vi"("错误输入"=w253, "motor"=w237, "com in"=w254) -> ("错误输出"=w189:errorcluster, "Pisotion"=w191:i32, "com out"=w190:refnum<visa-resource-name>)
            n113 = call "TMCM351-getSpeed.vi"("错误输入"=w189, "com in"=w190) -> ("错误输出"=w169:errorcluster, "Motion Done"=w157:bool, "com out"=w170:refnum<visa-resource-name>)  [unwired: 2 in, 1 out]
            n114 = call "pic_Limit.vi"("错误输入"=w169, "com in"=w170) -> ("错误输出"=w167:errorcluster, "Limit out"=w166:bool[], "com out"=w168:refnum<visa-resource-name>)  [unwired: 1 in]
            n115 = call "GetPosition.vi"("CmdLib In"=w185, "DeviceKey In"=w184, "Device Address In"=w183, "Motor"=w177, "error in (no error)"=w182) -> ("CmdLib Out"=w175:refnum<k24>, "Position"=w171:i32, "error out"=w174:errorcluster)  [unwired: 6 in, 2 out]
            n116 = Compound Arithmetic op=AND ("复合运算")(w223, w222, w158, w157) -> (→"执行":bool)
            n117 = Index Array(array=w166, index #1=0 ("索引")) -> (element #1=→"pic1Left":bool, element #2=→"pic1Right":bool, element #3=→"pic2Left":bool, element #4=→"pic2Right":bool, element #5=→"pic3Left":bool, element #6=→"pic3Right":bool)  [unwired: 5 in]
            n118 = Format Value(format string="X\\t%d" ("格式字符串"), value (0)=w194) -> (output string=w247:string)  [unwired: 1 in]
            n119 = Format Value(format string="Y\\t%d" ("格式字符串"), value (0)=w195) -> (output string=w246:string)  [unwired: 1 in]
            n120 = Format Value(format string="Z\\t%d" ("格式字符串"), value (0)=w191) -> (output string=w245:string)  [unwired: 1 in]
            n121 = Format Value(format string="P1\\t%d" ("格式字符串"), value (0)=w227) -> (output string=w244:string)  [unwired: 1 in]
            n122 = Format Value(format string="P2\\t%d" ("格式字符串"), value (0)=w226) -> (output string=w243:string)  [unwired: 1 in]
            n123 = Format Value(format string="P3\\t%d" ("格式字符串"), value (0)=w171) -> (output string=w172:string)  [unwired: 1 in]
            n124 = local write "CH3 当前位置"(w171) -> ()
            n125 = Build Array(w247, w246, w245, w244, w243, w172) -> (→"当前位置":string[])
          }
          event "CH1启动": Value Change {
            # "大于零右转"
            n126 = event-data() -> ()  [unwired: 1 in, 6 out]
            n127 = local read "CH1 运动步数"() -> (w267:i32)
            n128 = flat-sequence {
              tunnel: w276 -> [w283]
              tunnel: w275 -> [w282]
              tunnel: w267 -> [w280]
              tunnel: [w281] -> w272
              tunnel: [w277] -> w269
              tunnel: [w286] -> w274
              tunnel: w272 -> [w286]
              tunnel: [w284] -> w268
              tunnel: w269 -> [w284]
              frame #0 {
                n129 = call "go_one_step.vi"("error in"=w282, "Step"=w280, "Motor"=1, "CmdLib In"=w283) -> ("error out"=w281:errorcluster, "Position"=w278:i32, "CmdLib Out"=w277:refnum<k24>)  [unwired: 1 in]
                n130 = local write "CH1 当前位置"(w278) -> ()
              }
              frame #1 {
                w285 = FALSE ("制动")
                n131 = local write "制动"(w285) -> ()
                n132 = local write "CH1启动"(w285) -> ()
              }
            }
            n133 = Greater Than 0?(x=w267) -> (x > 0?=→"P1 右":bool)
          }
          event "P1 归0": Value Change {
            n134 = event-data() -> ()  [unwired: 1 in, 6 out]
            n135 = local read "CH1 当前位置"() -> (w298:i32)
            n136 = Multiply(x=w298, y=-1) -> (x*y=w296:i32)
            n137 = flat-sequence {
              tunnel: w296 -> [w305]
              tunnel: w295 -> [w304]
              tunnel: w294 -> [w303]
              tunnel: [w302] -> w291
              tunnel: [w299] -> w290
              tunnel: [w308] -> w292
              tunnel: w291 -> [w308]
              tunnel: [w306] -> _
              tunnel: w290 -> [w306]
              tunnel: [w306] -> w289
              frame #0 {
                n138 = call "go_one_step.vi"("error in"=w303, "Step"=w305, "Motor"=1, "CmdLib In"=w304) -> ("error out"=w302:errorcluster, "Position"=w300:i32, "CmdLib Out"=w299:refnum<k24>)  [unwired: 1 in]
                n139 = local write "CH1 当前位置"(w300) -> ()
              }
              frame #1 {
                w307 = FALSE ("制动")
                n140 = local write "P1 归0"(w307) -> ()
                n141 = local write "制动"(w307) -> ()
              }
            }
          }
          event "CH2启动": Value Change {
            n142 = event-data() -> ()  [unwired: 1 in, 6 out]
            n143 = local read "CH2 运动步数"() -> (w310:i32)
            n144 = flat-sequence {
              tunnel: w319 -> [w326]
              tunnel: w317 -> [w324]
              tunnel: [w325] -> w315
              tunnel: [w321] -> w312
              tunnel: w310 -> [w320]
              tunnel: [w329] -> w318
              tunnel: w315 -> [w329]
              tunnel: [w327] -> w311
              tunnel: w312 -> [w327]
              frame #0 {
                n145 = call "go_one_step.vi"("error in"=w324, "Step"=w320, "Motor"=2, "CmdLib In"=w326) -> ("error out"=w325:errorcluster, "Position"=w322:i32, "CmdLib Out"=w321:refnum<k24>)  [unwired: 1 in]
                n146 = local write "CH2 当前位置"(w322) -> ()
              }
              frame #1 {
                w328 = FALSE
                n147 = local write "CH2启动"(w328) -> ()
                n148 = local write "制动"(w328) -> ()
              }
            }
            n149 = Greater Than 0?(x=w310) -> (x > 0?=→"P2 右":bool)
          }
          event "CH3启动": Value Change {
            n150 = event-data() -> ()  [unwired: 1 in, 6 out]
            n151 = flat-sequence {
              tunnel: w338 -> [w346]
              tunnel: w337 -> [w345]
              tunnel: [w343] -> w332
              tunnel: [w341] -> w331
              tunnel: [w348] -> w335
              tunnel: [w349] -> w336
              tunnel: w332 -> [w349]
              tunnel: w331 -> [w348]
              frame #0 {
                n152 = local read "CH3 运动步数"() -> (w340:i32)
                n153 = call "go_one_step.vi"("error in"=w345, "Step"=w340, "Motor"=3, "CmdLib In"=w346) -> ("error out"=w341:errorcluster, "Position"=w342:i32, "CmdLib Out"=w343:refnum<k24>)  [unwired: 1 in]
                n154 = Greater Than 0?(x=w340) -> (x > 0?=→"P3右":bool)
                n155 = local write "CH3 当前位置"(w342) -> ()
              }
              frame #1 {
                w347 = FALSE
                n156 = local write "CH3启动"(w347) -> ()
                n157 = local write "制动"(w347) -> ()
              }
            }
          }
          event "P2归0": Value Change {
            n158 = event-data() -> ()  [unwired: 1 in, 6 out]
            n159 = local read "CH2 当前位置"() -> (w360:i32)
            n160 = Multiply(x=w360, y=-1) -> (x*y=w358:i32)
            n161 = flat-sequence {
              tunnel: w358 -> [w367]
              tunnel: w357 -> [w366]
              tunnel: w356 -> [w365]
              tunnel: [w364] -> w353
              tunnel: [w361] -> w352
              tunnel: [w369] -> w355
              tunnel: w353 -> [w369]
              frame #0 {
                n162 = call "go_one_step.vi"("error in"=w365, "Step"=w367, "Motor"=2, "CmdLib In"=w366) -> ("error out"=w364:errorcluster, "Position"=w362:i32, "CmdLib Out"=w361:refnum<k24>)  [unwired: 1 in]
                n163 = local write "CH2 当前位置"(w362) -> ()
              }
              frame #1 {
                w368 = FALSE ("制动")
                n164 = local write "P2归0"(w368) -> ()
                n165 = local write "制动"(w368) -> ()
              }
            }
          }
          event "P3归0": Value Change {
            n166 = event-data() -> ()  [unwired: 1 in, 6 out]
            n167 = local read "CH3 当前位置"() -> (w379:i32)
            n168 = Multiply(x=w379, y=-1) -> (x*y=w378:i32)
            n169 = flat-sequence {
              tunnel: w378 -> [w387]
              tunnel: w376 -> [w386]
              tunnel: w375 -> [w385]
              tunnel: [w384] -> w380
              tunnel: [w381] -> w372
              tunnel: w380 -> [w388]
              tunnel: [w388] -> w374
              frame #0 {
                n170 = call "go_one_step.vi"("error in"=w385, "Step"=w387, "Motor"=3, "CmdLib In"=w386) -> ("error out"=w384:errorcluster, "Position"=w382:i32, "CmdLib Out"=w381:refnum<k24>)  [unwired: 1 in]
                n171 = local write "CH3 当前位置"(w382) -> ()
              }
              frame #1 {
                w389 = FALSE ("制动")
                n172 = local write "P3归0"(w389) -> ()
                n173 = local write "制动"(w389) -> ()
              }
            }
          }
          event "制动": Value Change {
            w396 = u8 2 items=["x", "y", "z"] ("motor")
            w399 = u8 1 items=["x", "y", "z"] ("motor")
            w402 = u8 0 items=["x", "y", "z"] ("motor")
            (unwired) 2 ("Motor")
            (unwired) 1 ("Motor")
            n174 = event-data() -> ("OldVal"=w390:bool)  [unwired: 1 in, 5 out]
            n175 = local write "制动"(w390) -> ()
            n176 = call "TMCM351-STOP.vi"("错误输入"=w403, "motor"=w402, "com in"=w404) -> ("错误输出"=w400:errorcluster, "com out"=w401:refnum<visa-resource-name>)
            n177 = global read "Verbal.vi" "Device Address"() -> (w393:i32)
            n178 = global read "Verbal.vi" "DeviceKey"() -> (w405:string)
            n179 = call "TMCM351-STOP.vi"("错误输入"=w400, "motor"=w399, "com in"=w401) -> ("错误输出"=w397:errorcluster, "com out"=w398:refnum<visa-resource-name>)
            n180 = call "AbortMotion.vi"("error in (no error)"=w407, "Device Address In"=w393, "DeviceKey In"=w405, "CmdLib In"=w406) -> ("error out"=w392:errorcluster, "CmdLib Out"=w391:refnum<k24>)  [unwired: 2 out]
            n181 = call "TMCM351-STOP.vi"("错误输入"=w397, "motor"=w396, "com in"=w398) -> ("错误输出"=w394:errorcluster, "com out"=w395:refnum<visa-resource-name>)
          }
          event Application Instance Close {
            w414 = u8 2 items=["x", "y", "z"] ("motor")
            w415 = u8 1 items=["x", "y", "z"] ("motor")
            w420 = u8 0 items=["x", "y", "z"] ("motor")
            n182 = event-data() -> ()  [unwired: 1 in, 4 out]
            n183 = call "Shutdown.vi"("error in (no error)"=w423, "CmdLib In"=w424) -> ("error out"=w422:errorcluster, "CmdLib Out"=w409:refnum<k24>)  [unwired: 4 in]
            n184 = call "TMCM351-STOP.vi"("错误输入"=w412, "motor"=w420, "com in"=w413) -> ("错误输出"=w419:errorcluster, "com out"=w418:refnum<visa-resource-name>)
            n185 = call "TMCM351-STOP.vi"("错误输入"=w419, "motor"=w415, "com in"=w418) -> ("错误输出"=w417:errorcluster, "com out"=w416:refnum<visa-resource-name>)
            n186 = call "TMCM351-STOP.vi"("错误输入"=w417, "motor"=w414, "com in"=w416) -> ("错误输出"=w410:errorcluster, "com out"=w411:refnum<visa-resource-name>)
          }
          event "结束": Value Change {
            w436 = u8 2 items=["x", "y", "z"] ("motor")
            w437 = u8 1 items=["x", "y", "z"] ("motor")
            w438 = u8 0 items=["x", "y", "z"] ("motor")
            n187 = event-data() -> ()  [unwired: 1 in, 6 out]
            n188 = call "Shutdown.vi"("error in (no error)"=w430, "CmdLib In"=w431) -> ("error out"=w426:errorcluster, "CmdLib Out"=w427:refnum<k24>)  [unwired: 4 in]
            n189 = call "TMCM351-STOP.vi"("错误输入"=w432, "motor"=w438, "com in"=w435) -> ("错误输出"=w439:errorcluster, "com out"=w434:refnum<visa-resource-name>)
            n190 = call "TMCM351-STOP.vi"("错误输入"=w439, "motor"=w437, "com in"=w434) -> ("错误输出"=w440:errorcluster, "com out"=w433:refnum<visa-resource-name>)
            n191 = call "TMCM351-STOP.vi"("错误输入"=w440, "motor"=w436, "com in"=w433) -> ("错误输出"=w428:errorcluster, "com out"=w429:refnum<visa-resource-name>)
          }
          event Panel Close {
            w445 = u8 2 items=["x", "y", "z"] ("motor")
            w446 = u8 1 items=["x", "y", "z"] ("motor")
            w451 = u8 0 items=["x", "y", "z"] ("motor")
            n192 = event-data() -> ()  [unwired: 1 in, 4 out]
            n193 = call "Shutdown.vi"("error in (no error)"=w455, "CmdLib In"=w456) -> ("error out"=w454:errorcluster, "CmdLib Out"=w452:refnum<k24>)  [unwired: 4 in]
            n194 = call "TMCM351-STOP.vi"("错误输入"=w443, "motor"=w451, "com in"=w444) -> ("错误输出"=w450:errorcluster, "com out"=w449:refnum<visa-resource-name>)
            n195 = call "TMCM351-STOP.vi"("错误输入"=w450, "motor"=w446, "com in"=w449) -> ("错误输出"=w448:errorcluster, "com out"=w447:refnum<visa-resource-name>)
            n196 = call "TMCM351-STOP.vi"("错误输入"=w448, "motor"=w445, "com in"=w447) -> ("错误输出"=w441:errorcluster, "com out"=w442:refnum<visa-resource-name>)
          }
          event "X 启动": Value Change {
            w467 = u8 0 items=["x", "y", "z"] ("motor")
            n197 = event-data() -> ("CtlRef"=w458:refnum<vi>, "OldVal"=w457:bool)  [unwired: 1 in, 4 out]
            n198 = property class="Bool (严格)"(reference=w458, "Value"=w457) -> ()  [unwired: 1 in, 2 out]
            n199 = call "TMCM351-Step.vi"("错误输入"=w465, "Step"="Step X", "motor"=w467, "com in"=w466) -> ("错误输出"=w462:errorcluster, "com out"=w463:refnum<visa-resource-name>)  [unwired: 2 in]
          }
          event "Y 启动": Value Change {
            w478 = u8 1 items=["x", "y", "z"] ("motor")
            n200 = event-data() -> ("CtlRef"=w469:refnum<vi>, "OldVal"=w468:bool)  [unwired: 1 in, 4 out]
            n201 = property class="Bool (严格)"(reference=w469, "Value"=w468) -> ()  [unwired: 1 in, 2 out]
            n202 = call "TMCM351-Step.vi"("错误输入"=w476, "Step"="Step Y", "motor"=w478, "com in"=w477) -> ("错误输出"=w471:errorcluster, "com out"=w472:refnum<visa-resource-name>)  [unwired: 2 in]
          }
          event "Z 启动": Value Change {
            w488 = u8 2 items=["x", "y", "z"] ("motor")
            n203 = event-data() -> ("CtlRef"=w480:refnum<vi>, "OldVal"=w479:bool)  [unwired: 1 in, 4 out]
            n204 = property class="Bool (严格)"(reference=w480, "Value"=w479) -> ()  [unwired: 1 in, 2 out]
            n205 = call "TMCM351-Step.vi"("错误输入"=w487, "Step"="Step Z", "motor"=w488, "com in"=w489) -> ("错误输出"=w482:errorcluster, "com out"=w483:refnum<visa-resource-name>)  [unwired: 2 in]
          }
          event "X 归0": Value Change {
            w490 = u8 0 items=["x", "y", "z"] ("motor")
            # "判断当前位置，大于0反转，小于0正转"
            n206 = event-data() -> ("CtlRef"=w496:refnum<vi>, "OldVal"=w495:bool)  [unwired: 1 in, 4 out]
            n207 = global write "Verbal.vi" "0位"(u8 1 ("0位")) -> ()
            n208 = property class="Bool (严格)"(reference=w496, "Value"=w495) -> ()  [unwired: 1 in, 2 out]
            n209 = call "TMCM1021_goRef.vi"("错误输入"=w491, "motor"=w490, "com in"=w494) -> ("错误输出"=w492:errorcluster, "com out"=w493:refnum<visa-resource-name>)
          }
          event "Y 归0": Value Change {
            w503 = u8 1 items=["x", "y", "z"] ("motor")
            n210 = event-data() -> ("CtlRef"=w507:refnum<vi>, "OldVal"=w506:bool)  [unwired: 1 in, 4 out]
            n211 = global write "Verbal.vi" "0位"(u8 2 ("0位")) -> ()
            n212 = property class="Bool (严格)"(reference=w507, "Value"=w506) -> ()  [unwired: 1 in, 2 out]
            n213 = call "TMCM1021_goRef.vi"("错误输入"=w504, "motor"=w503, "com in"=w505) -> ("错误输出"=w501:errorcluster, "com out"=w502:refnum<visa-resource-name>)
          }
          event "Z 归0": Value Change {
            w515 = u8 2 items=["x", "y", "z"] ("motor")
            n214 = event-data() -> ("CtlRef"=w519:refnum<vi>, "OldVal"=w518:bool)  [unwired: 1 in, 4 out]
            n215 = global write "Verbal.vi" "0位"(u8 3 ("0位")) -> ()
            n216 = property class="Bool (严格)"(reference=w519, "Value"=w518) -> ()  [unwired: 1 in, 2 out]
            n217 = call "TMCM1021_goRef.vi"("错误输入"=w516, "motor"=w515, "com in"=w517) -> ("错误输出"=w513:errorcluster, "com out"=w514:refnum<visa-resource-name>)
          }
          event "X 连续正转": Value Change {
            w530 = u8 0 items=["x", "y", "z"] ("motor")
            n218 = event-data() -> ("CtlRef"=w527:refnum<vi>, "OldVal"=w526:bool)  [unwired: 1 in, 4 out]
            n219 = property class="Bool (严格)"(reference=w527, "Value"=w526) -> ()  [unwired: 1 in, 2 out]
            n220 = global read "Verbal.vi" "speed step"() -> (w532)
            n221 = call "TMCM351-rotate.vi"("motor"=w530, "错误输入"=w533, "正转？"=TRUE, "Speed"=w532, "com in"=w534) -> ("错误输出"=w528:errorcluster, "com out"=w529:refnum<visa-resource-name>)  [unwired: 2 in]
          }
          event "Y 连续正转": Value Change {
            w544 = u8 1 items=["x", "y", "z"] ("motor")
            n222 = event-data() -> ("CtlRef"=w539:refnum<vi>, "OldVal"=w538:bool)  [unwired: 1 in, 4 out]
            n223 = property class="Bool (严格)"(reference=w539, "Value"=w538) -> ()  [unwired: 1 in, 2 out]
            n224 = global read "Verbal.vi" "speed step"() -> (w546)
            n225 = call "TMCM351-rotate.vi"("motor"=w544, "错误输入"=w542, "正转？"=TRUE, "Speed"=w546, "com in"=w543) -> ("错误输出"=w540:errorcluster, "com out"=w541:refnum<visa-resource-name>)  [unwired: 2 in]
          }
          event "Z 连续正转": Value Change {
            w556 = u8 2 items=["x", "y", "z"] ("motor")
            n226 = event-data() -> ("CtlRef"=w551:refnum<vi>, "OldVal"=w550:bool)  [unwired: 1 in, 4 out]
            n227 = property class="Bool (严格)"(reference=w551, "Value"=w550) -> ()  [unwired: 1 in, 2 out]
            n228 = global read "Verbal.vi" "speed step"() -> (w558)
            n229 = call "TMCM351-rotate.vi"("motor"=w556, "错误输入"=w554, "正转？"=TRUE, "Speed"=w558, "com in"=w555) -> ("错误输出"=w552:errorcluster, "com out"=w553:refnum<visa-resource-name>)  [unwired: 2 in]
          }
          event "X连续反转": Value Change {
            w568 = u8 0 items=["x", "y", "z"] ("motor")
            n230 = event-data() -> ("CtlRef"=w563:refnum<vi>, "OldVal"=w562:bool)  [unwired: 1 in, 4 out]
            n231 = property class="Bool (严格)"(reference=w563, "Value"=w562) -> ()  [unwired: 1 in, 2 out]
            n232 = global read "Verbal.vi" "speed step"() -> (w570)
            n233 = call "TMCM351-rotate.vi"("motor"=w568, "错误输入"=w566, "正转？"=FALSE, "Speed"=w570, "com in"=w567) -> ("错误输出"=w564:errorcluster, "com out"=w565:refnum<visa-resource-name>)  [unwired: 2 in]
          }
          event "Y 连续反转": Value Change {
            w581 = u8 1 items=["x", "y", "z"] ("motor")
            n234 = event-data() -> ("CtlRef"=w575:refnum<vi>, "OldVal"=w574:bool)  [unwired: 1 in, 4 out]
            n235 = property class="Bool (严格)"(reference=w575, "Value"=w574) -> ()  [unwired: 1 in, 2 out]
            n236 = global read "Verbal.vi" "speed step"() -> (w582)
            n237 = call "TMCM351-rotate.vi"("motor"=w581, "错误输入"=w578, "正转？"=FALSE, "Speed"=w582, "com in"=w579) -> ("错误输出"=w576:errorcluster, "com out"=w577:refnum<visa-resource-name>)  [unwired: 2 in]
          }
          event "Z 连续反转": Value Change {
            w592 = u8 2 items=["x", "y", "z"] ("motor")
            n238 = event-data() -> ("CtlRef"=w587:refnum<vi>, "OldVal"=w586:bool)  [unwired: 1 in, 4 out]
            n239 = property class="Bool (严格)"(reference=w587, "Value"=w586) -> ()  [unwired: 1 in, 2 out]
            n240 = global read "Verbal.vi" "speed step"() -> (w594)
            n241 = call "TMCM351-rotate.vi"("motor"=w592, "错误输入"=w590, "正转？"=FALSE, "Speed"=w594, "com in"=w591) -> ("错误输出"=w588:errorcluster, "com out"=w589:refnum<visa-resource-name>)  [unwired: 2 in]
          }
          event "X jog": Value Change {
            w599 = u8 0 items=["x", "y", "z"] ("motor")
            n242 = event-data() -> ("CtlRef"=w605:refnum<vi>, "OldVal"=w604:bool)  [unwired: 1 in, 4 out]
            n243 = property class="Bool (严格)"(reference=w605, "Value"=w604) -> ()  [unwired: 1 in, 2 out]
            n244 = local read "X设定位置"() -> (w598:i32)
            n245 = call "TMCM351-goJog.vi"("错误输入"=w602, "step in"=w598, "motor"=w599, "com in"=w603) -> ("错误输出"=w600:errorcluster, "com out"=w601:refnum<visa-resource-name>)  [unwired: 2 in]
          }
          event "Yjog": Value Change {
            w612 = u8 1 items=["x", "y", "z"] ("motor")
            n246 = event-data() -> ("CtlRef"=w616:refnum<vi>, "OldVal"=w615:bool)  [unwired: 1 in, 4 out]
            n247 = property class="Bool (严格)"(reference=w616, "Value"=w615) -> ()  [unwired: 1 in, 2 out]
            n248 = local read "Y设定位置"() -> (w611:i32)
            n249 = call "TMCM351-goJog.vi"("错误输入"=w613, "step in"=w611, "motor"=w612, "com in"=w614) -> ("错误输出"=w609:errorcluster, "com out"=w610:refnum<visa-resource-name>)  [unwired: 2 in]
          }
          event "Zjog": Value Change {
            w623 = u8 2 items=["x", "y", "z"] ("motor")
            n250 = event-data() -> ("CtlRef"=w627:refnum<vi>, "OldVal"=w626:bool)  [unwired: 1 in, 4 out]
            n251 = property class="Bool (严格)"(reference=w627, "Value"=w626) -> ()  [unwired: 1 in, 2 out]
            n252 = local read "Z设定位置"() -> (w622:i32)
            n253 = call "TMCM351-goJog.vi"("错误输入"=w624, "step in"=w622, "motor"=w623, "com in"=w625) -> ("错误输出"=w620:errorcluster, "com out"=w621:refnum<visa-resource-name>)  [unwired: 2 in]
          }
          event "P1jog": Value Change {
            n254 = event-data() -> ("CtlRef"=w640:refnum<vi>, "OldVal"=w639:bool)  [unwired: 1 in, 4 out]
            n255 = property class="Bool (严格)"(reference=w640, "Value"=w639) -> ()  [unwired: 1 in, 2 out]
            n256 = global read "Verbal.vi" "Device Address"() -> (w636:i32)
            n257 = local read "P1设定位置"() -> (w634:i32)
            n258 = global read "Verbal.vi" "DeviceKey"() -> (w637:string)
            n259 = call "AbsoluteMove.vi"("CmdLib In"=w638, "DeviceKey In"=w637, "Device Address In"=w636, "Motor"=1, "Target Pos"=w634, "error in (no error)"=w633) -> ("CmdLib Out"=w632:refnum<k24>, "error out"=w631:errorcluster)  [unwired: 10 in, 2 out]
          }
          event "P2 jog": Value Change {
            n260 = event-data() -> ("CtlRef"=w653:refnum<vi>, "OldVal"=w652:bool)  [unwired: 1 in, 4 out]
            n261 = property class="Bool (严格)"(reference=w653, "Value"=w652) -> ()  [unwired: 1 in, 2 out]
            n262 = global read "Verbal.vi" "Device Address"() -> (w649:i32)
            n263 = global read "Verbal.vi" "DeviceKey"() -> (w650:string)
            n264 = local read "P2设定位置"() -> (w647:i32)
            n265 = call "AbsoluteMove.vi"("CmdLib In"=w651, "DeviceKey In"=w650, "Device Address In"=w649, "Motor"=2, "Target Pos"=w647, "error in (no error)"=w646) -> ("CmdLib Out"=w645:refnum<k24>, "error out"=w644:errorcluster)  [unwired: 10 in, 2 out]
          }
        }
      }
    }
  }
  n266 = call "Shutdown.vi"("error in (no error)"=w3, "CmdLib In"=w4) -> ("error out"=w5:errorcluster, "CmdLib Out"=w6:refnum<k24>)  [unwired: 4 in]
  n267 = call "CloseDevice.vi"("error in"=w5, "CmdLib In"=w6) -> ("error out"=→"error out":errorcluster)  [unwired: 8 in, 1 out]
  n268 = call "TMCM351-STOP.vi"("错误输入"=w13, "motor"=w12, "com in"=w14) -> ("错误输出"=w17:errorcluster, "com out"=w18:refnum<visa-resource-name>)
  n269 = call "TMCM351-STOP.vi"("错误输入"=w17, "motor"=w11, "com in"=w18) -> ("错误输出"=w15:errorcluster, "com out"=w16:refnum<visa-resource-name>)
  n270 = call "TMCM351-STOP.vi"("错误输入"=w15, "motor"=w10, "com in"=w16) -> ("错误输出"=w8:errorcluster, "com out"=w9:refnum<visa-resource-name>)
  n271 = call "TMCM351-STOPexe.vi"("错误输入"=w8, "com in"=w9) -> ("错误输出"=w19:errorcluster, "com out"=w20:refnum<visa-resource-name>)
  n272 = VISA Close(VISA resource name=w20, error in (no error)=w19) -> ()  [unwired: 1 out]
